vi "Shooter at Speed.vi"(9 "Shot Error Thresh":dbl=5.0, 10 "Shooter RPM":dbl, 11 "Target Velocity":dbl) -> (3 "Shooter at Speed":bool)   [LabVIEW 2015]
panel:
  # "in rpm"
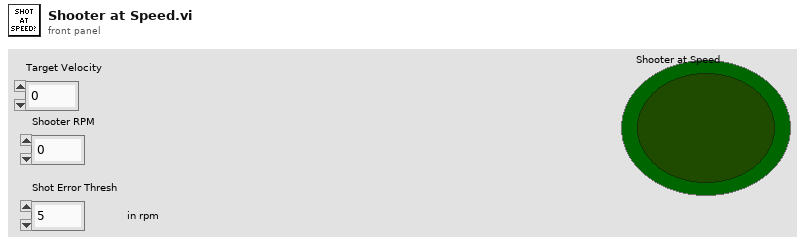
[diagram p1: front panel]
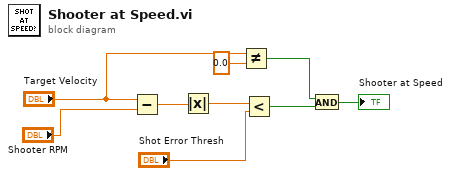
[diagram p0: block diagram]
diagram:
  n1 = Subtract(x="Target Velocity", y="Shooter RPM") -> (x-y=w8:dbl)
  n2 = Absolute Value(x=w8) -> (abs(x)=w7:dbl)
  n3 = Not Equal?(x="Target Velocity", y=0.0) -> (x != y?=w3:bool)
  n4 = Less?(x=w7, y="Shot Error Thresh") -> (x < y?=w2:bool)
  n5 = And(x=w3, y=w2) -> (x .and. y?=→"Shooter at Speed":bool)
